vi "Send Set Sensor COM Port.vi"(7 "Priority":T1=enum."Normal" caption="Message Priority (Normal)", 8 "error in (no error)":errorcluster, 10 "COM Port":refnum<visa-resource-name>, 11 "Message Enqueuer in":refnum<class "Message Enqueuer.lvclass">) -> (0 "error out":errorcluster, 3 "Message Enqueuer out":refnum<class "Message Enqueuer.lvclass">)   [LabVIEW 2018, in "Sensor.lvlib" / "Set Sensor COM Port Msg.lvclass"]
doc: "Sends the <b>Sensor.lvlib:Set Sensor COM Port Msg.lvclass</b> message.\n\nThis message will call <b>Set Sensor COM Port.vi</b> on the <b>Sensor.lvlib:Sensor.lvclass</b> actor.\n\n<b>Set Sensor COM Port.vi Description</b>"
uses:
  Set Sensor COM Port Msg.lvclass
  <vilib>/ActorFramework/Message Enqueuer/Message Enqueuer.lvclass
  <vilib>/ActorFramework/Message Enqueuer/Message Priority.ctl
  C:/Program Files (x86)/National Instruments/LabVIEW 2018/vi.lib/ActorFramework/Message/Message.lvclass
  Set Sensor COM Port Msg.lvclass/Set Sensor COM Port Msg.ctl
  <vilib>/ActorFramework/Message Enqueuer/Message Enqueuer.lvclass/Message Enqueuer.ctl
  <vilib>/ActorFramework/Message Priority Queue/Priority Enqueue.vi
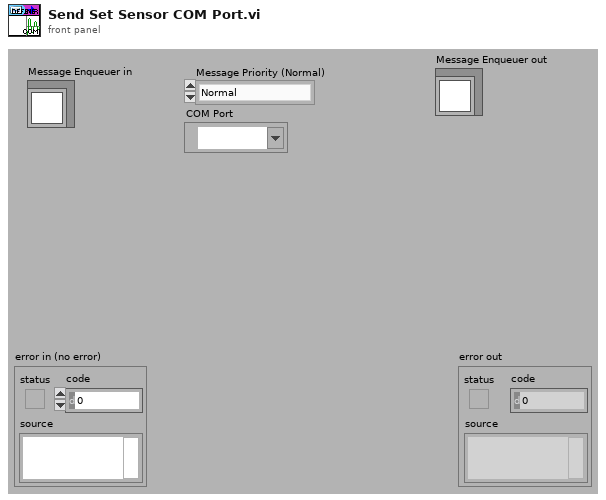
[diagram p1: front panel]
types:
  T1 = typedef "Actor Framework.lvlib/Message Enqueuer.lvclass/Message Priority.ctl" = enum16{"Low", "Normal", "High"}
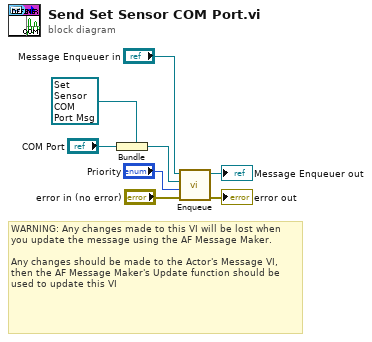
[diagram p0: block diagram]
diagram:
  # "WARNING: Any changes made to this VI will be lost when you update the message using the AF Message Maker.\n\nAny changes should be made to the Actor's Message VI, then the AF Message Maker's Update function should be used to update this VI"
  n1 = Bundle(cluster=refnum<class "Set Sensor COM Port Msg.lvclass"> refnum ("Sensor.lvlib:Set Sensor COM Port Msg.lvclass"), "COM Port") -> (w4:refnum<class "Set Sensor COM Port Msg.lvclass">)
  n2 = call <vilib>:"Enqueue.vi"("error in (no error)"="error in (no error)", "Message Priority (Normal)"="Priority", "Message"=w4, "Message Enqueuer in"="Message Enqueuer in") -> ("error out"=→"error out":errorcluster, "Message Enqueuer out"=→"Message Enqueuer out":refnum<class "Message Enqueuer.lvclass">)  [unwired: 6 in]
